vi "Read Voltage Power Supply.vi"(10 "Channel":enum16{"Positive", "Negative"}(ring), 11 "ADALM2000 Handler":u64 caption="Instrument Handle Out") -> (2 "Read Voltage":dbl(knob) scale=0.0..10.0, 3 "ADALM2000 Handler 2":u64 caption="Instrument Handle Out")   [LabVIEW 2022 SP3]
uses:
  libm2k_lv.dll
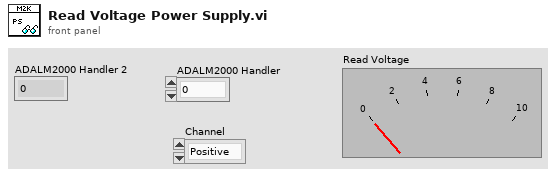
[diagram p1: front panel]
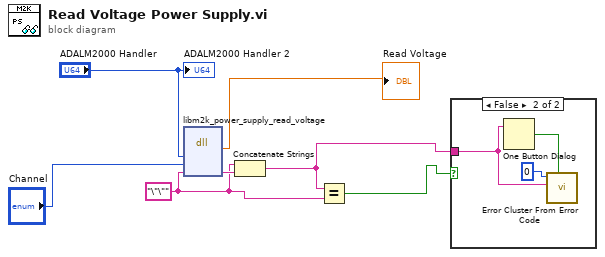
[diagram p0: block diagram]
diagram:
  w5 = "\"\""
  n1 = dll-call lib="libm2k_lv.*" fn="libm2k_power_supply_read_voltage"("instance"="ADALM2000 Handler", "chnIdx"="Channel", "err"=w5) -> ("return type"=→"Read Voltage":dbl, "err"=w7:string)  [unwired: 5 in, 2 out]
  n2 = Concatenate Strings(w5, w7) -> (w3:string)
  n3 = Equal?(x=w3, y=w5) -> (x = y?=w4:bool)
  n4 = case shown="False" w4 {
    tunnel: w3 -> [_ w8]
    frame True {
    }
    frame False {
      n5 = One Button Dialog(message=w8) -> (true=w10:bool)  [unwired: 1 in]
      n6 = call <vilib>:"Error Cluster From Error Code.vi"("show call chain? (False)"=w10, "error message (\"\")"=w8, "error code (0)"=0) -> ()  [unwired: 6 in, 1 out]
    }
  }
  "ADALM2000 Handler 2" <- "ADALM2000 Handler"
